vi "Manchester encoder.vi"(8 "Error In":errorcluster, 10 "Bit stream in":u8[](array[numeric])) -> (0 "error out":errorcluster {"code" format="Error %.0f"}, 2 "Bit stream out (Manchester encode)":u8[](array[numeric]))   [LabVIEW 2019]
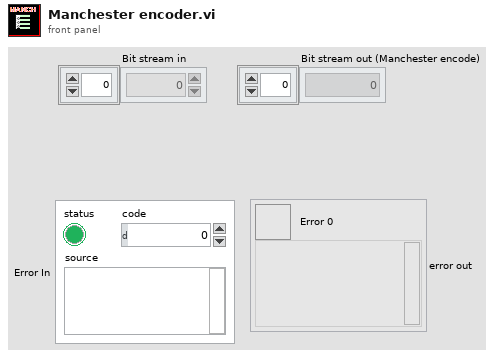
[diagram p1: front panel]
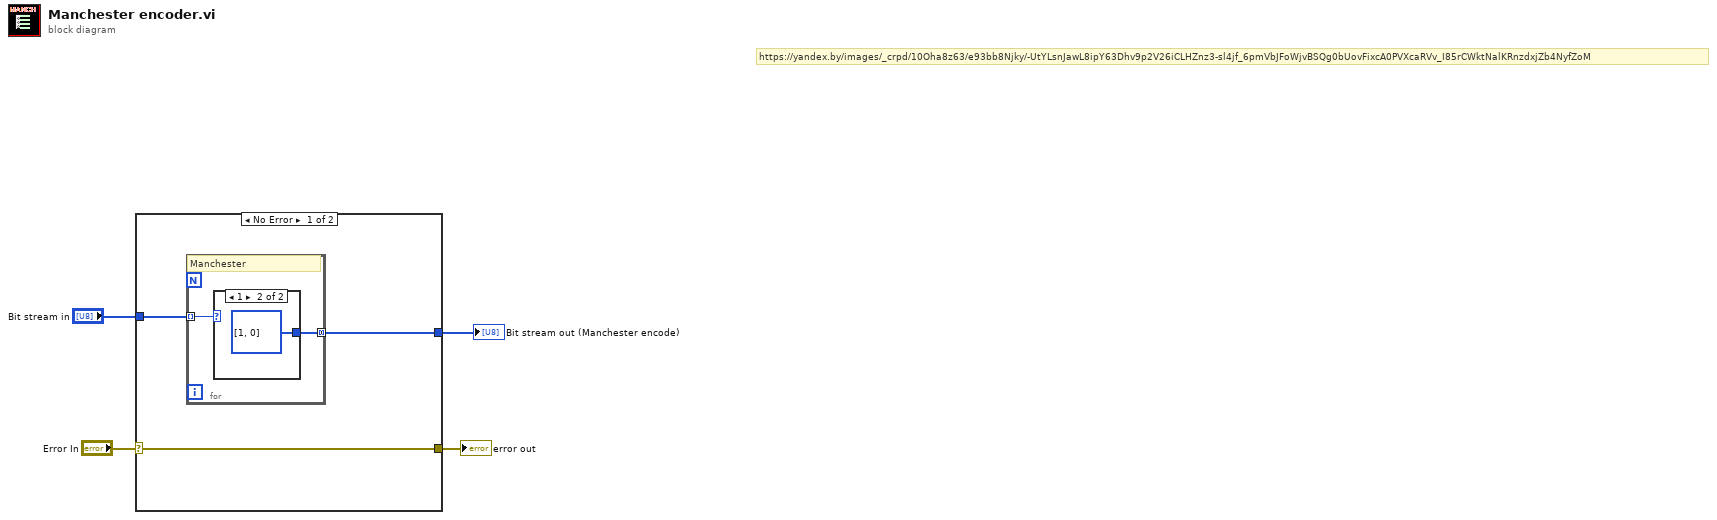
[diagram p0: block diagram]
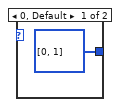
[diagram p2: hidden frame]
diagram:
  # "https://yandex.by/images/_crpd/10Oha8z63/e93bb8Njky/-UtYLsnJawL8ipY63Dhv9p2V26iCLHZnz3-sl4jf_6pmVbJFoWjvBSQg0bUovFixcA0PVXcaRVv_I85rCWktNalKRnzdxjZb4NyfZoM"
  n1 = case shown="No Error" "Error In" {
    selector: "Error In" -> [w5 w12]
    tunnel: "Bit stream in" -> [w7 _]
    tunnel: [w6 _] -> w3
    tunnel: [w5 w12] -> w1
    frame No Error {
      n2 = for {
        tunnel: w7 -> [w9] mode=indexing
        tunnel: [w8] -> w6 mode=concatenating
        # "Manchester"
        n3 = case shown="1" w9 {
          tunnel: [u8[] [0, 1] ("output array") u8[] [1, 0] ("output array")] -> w8
          frame 0, Default {
          }
          frame 1 {
          }
        }
      }
    }
    frame Error {
    }
  }
  "Bit stream out (Manchester encode)" <- w3
  "error out" <- w1
